vi "Write Running VI reference.vi"(8 "error in (no error)":errorcluster, 10 "Running VI reference":refnum<vi>, 11 "Fiber Auto Collimation panel in":refnum<class "Fiber Auto Collimation panel.lvclass">) -> (0 "error out":errorcluster, 3 "Fiber Auto Collimation panel out":refnum<class "Fiber Auto Collimation panel.lvclass">)   [LabVIEW 2018, in "Fiber Auto Collimation panel.lvclass"]
doc: "Writes a reference to the running VI of a panel.\n\nThis VI is private because it should only be called from the \"Register panel as running\" VI, which is used to keep track of which panels are running and which have terminated."
uses:
  Fiber Auto Collimation panel.lvclass
  Fiber Auto Collimation panel.lvclass/Fiber Auto Collimation panel.ctl
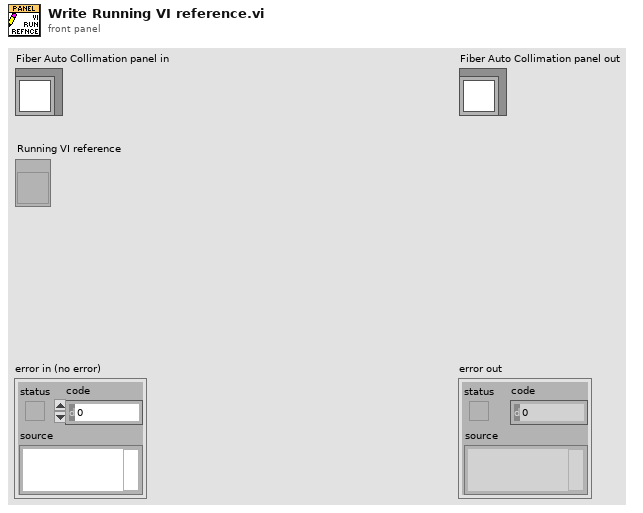
[diagram p1: front panel]
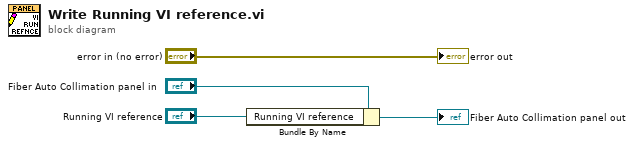
[diagram p0: block diagram]
diagram:
  n1 = Bundle By Name(cluster="Fiber Auto Collimation panel in", "Running VI reference"="Running VI reference") -> (→"Fiber Auto Collimation panel out":refnum<class "Fiber Auto Collimation panel.lvclass">)
  "error out" <- "error in (no error)"
